vi "AuMT8852B Instrument Status Register Query.vi"(8 "error in (no error)":errorcluster, 11 "VISA session":refnum<visa-resource-name>) -> (0 "error out":errorcluster, 2 "error code":i32, 3 "VISA session out":refnum<visa-resource-name>, 4 "Flags":T1, 6 "Value":i32)   [LabVIEW 2017]
doc: "Anritsu MT8852B Bluetooth Tester\n\nReturns an integer (0-255) containing information about the insrtument's status.\n\nBit 2 - Script or test completion - this bit is cleared when a test or script has started and is set on its completion.\nBit 1 - Disconnect - this bit is cleared when a connection has been made and set when the EUT is disconnected..\nBit 0 (least significant bit) - Connection - this bit is set when a connection has been made and cleared when the connection no longer exists.\n\nOUTPUTS\nFlags - meaning of each individual bit in the register.\nValue - integer value (0-255) of the register."
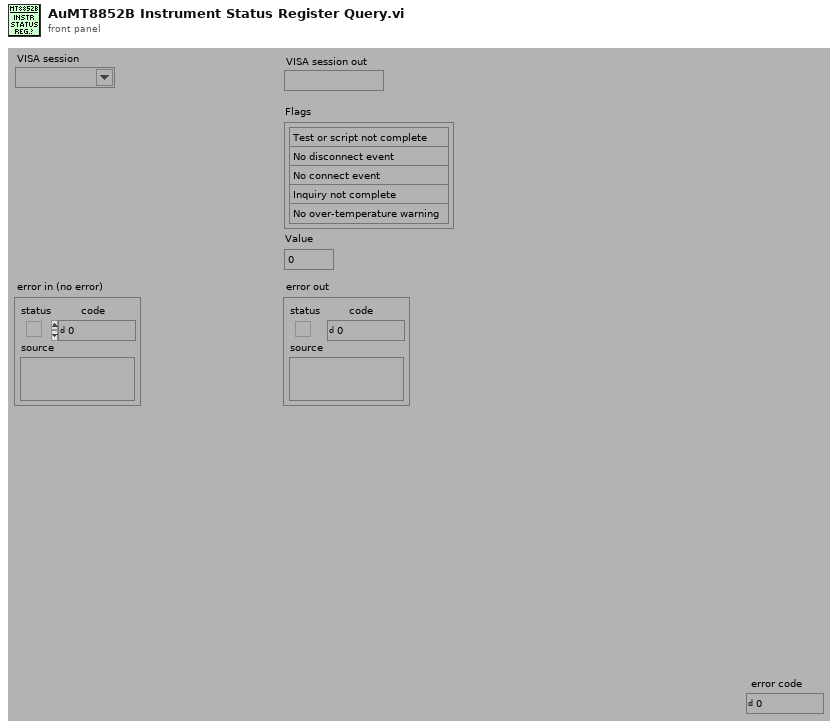
[diagram p1: front panel]
types:
  T1 = cluster{"Completion":enum16{"Test or script not complete", "Test or script complete"}, "Disconnect":enum16{"No disconnect event", "Disconnect event"}, "Connect":enum16{"No connect event", "Connect event"}, "Inquiry":enum16{"Inquiry not complete", "Inquiry complete"}, "Temperature":enum16{"No over-temperature warning", "Over-temperature warning"}}
  T2 = enum16{"Simulate", "Range check", "Cache", "Query instrument status"}
  T3 = cluster{"[0]":i16, "[1]":i16, "[2]":i16, "[3]":i16, "[4]":i16, "[5]":i16, "[6]":i16, "[7]":i16}
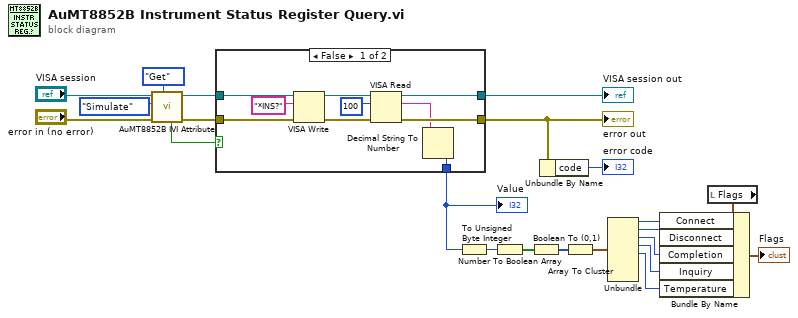
[diagram p0: block diagram]
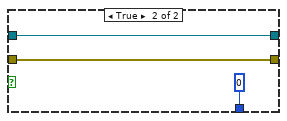
[diagram p2: hidden frame]
diagram:
  n1 = call <instrlib>:"AuMT8852B IVI Attribute.vi"("Set/Get (Set)"=enum16{"Set", "Get"}."Get", "error in (no error)"="error in (no error)", "Flag (Simulate)"=T2."Simulate", "VISA session"="VISA session") -> ("error out"=w18:errorcluster, "VISA session out"=w19:refnum<visa-resource-name>, "Value out"=w15:bool)  [unwired: 5 in]
  n2 = case shown="False" w15 {
    tunnel: [w26 w34] -> w3
    tunnel: [w27 w35] -> w20
    tunnel: w19 -> [w32 w35]
    tunnel: w18 -> [w31 w34]
    tunnel: [w23 0] -> w14
    frame False {
      n3 = VISA Write(VISA resource name=w32, write buffer="*INS?" ("write buffer (\"\")"), error in (no error)=w31) -> (VISA resource name out=w29:refnum<visa-resource-name>, error out=w28:errorcluster)  [unwired: 1 out]
      n4 = VISA Read(VISA resource name=w29, byte count=u32 100 ("byte count (0)"), error in (no error)=w28) -> (VISA resource name out=w27:refnum<visa-resource-name>, read buffer=w24:string, error out=w26:errorcluster)  [unwired: 1 out]
      n5 = Decimal String To Number(string=w24) -> (number=w23:i32)  [unwired: 2 in, 1 out]
    }
    frame True {
    }
  }
  "error out" <- w3
  "VISA session out" <- w20
  "Value" <- w14
  n6 = To Unsigned Byte Integer(number=w14) -> (unsigned 8bit integer=w13:u8)
  n7 = Number To Boolean Array(number=w13) -> (Boolean array=w12:bool[])
  n8 = Boolean To (0,1)(Boolean=w12) -> (0, 1=w11:i16[])
  n9 = Unbundle By Name(w3) -> ("code"=→"error code":i32)
  n10 = Array To Cluster(array=w11) -> (cluster=w10:T3)
  n11 = Unbundle(w10) -> ("[0]"=w7:i16, "[1]"=w6:i16, "[2]"=w5:i16, "[3]"=w2:i16, "[4]"=w1:i16)  [unwired: 3 out]
  n12 = local read "Flags"() -> (w9:T1)
  n13 = Bundle By Name(cluster=w9, "Connect"=w7, "Disconnect"=w6, "Completion"=w5, "Inquiry"=w2, "Temperature"=w1) -> (→"Flags":T1)
